vi "Test SimpleDependencyInspector API.vi"() -> ()   [LabVIEW 2019]
doc: "SimpleDependencyInspector API Tester."
uses:
  <vilib>/Utility/error.llb/DialogType.ctl
  arrow color--enum.ctl
  shape--enum.ctl
  SimpleDependencyInspector.lvlib
panel:
  in  "pattern":string[](array[string])=["*.lvlib", "*.lvclass"]
  out "Server Status":bool
  in  "Include vi.lib":bool
  in  "Folder to Inspect":path[](array[path])
  in  "Inspect Project Dependencies":bool
  out "last error":errorcluster
  in  "Show Diagram on Init":bool
  in  "Show Block Diagram":bool
  in  "Stop Module":bool
  in  "Start Module":bool
  in  "Hide Module Panel":bool
  in  "Show Module Panel":bool
  out "Status":string
  out "Module Running?":bool
  # "This VI tests the API for the Module."
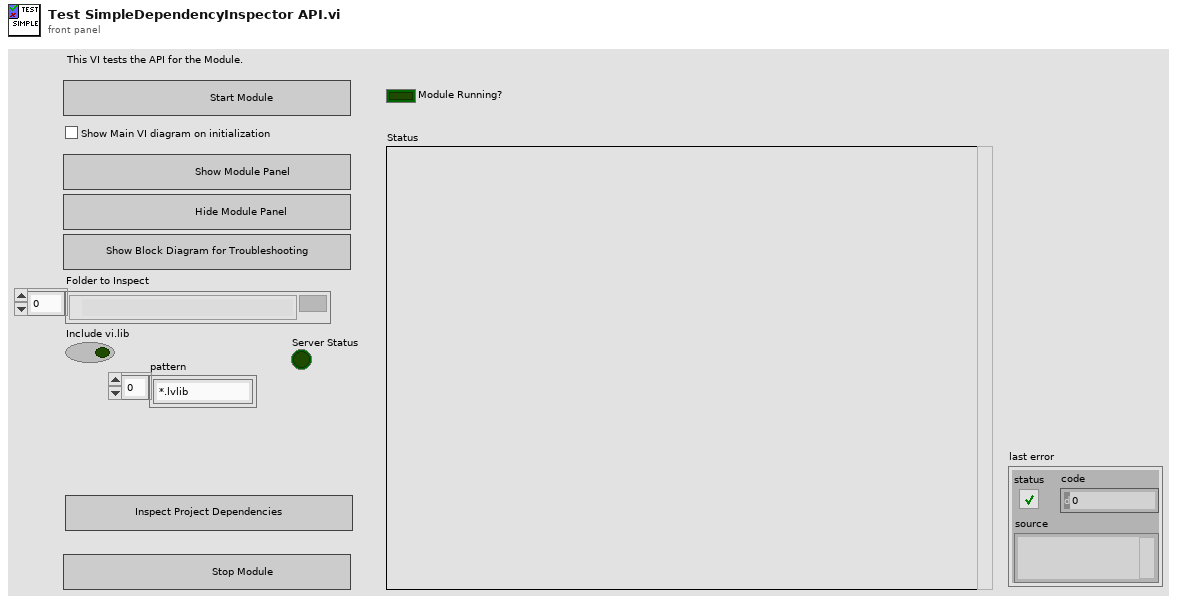
[diagram p1: front panel]
types:
  T1 = typedef "SimpleDependencyInspector.lvlib/Broadcast Events--cluster.ctl" = cluster{"Module Did Init":refnum<user-event>, "Status Updated":refnum<user-event>, "Error Reported":refnum<user-event>, "Module Did Stop":refnum<user-event>, "Update Module Execution Status":refnum<user-event>, "Server Status Updated":refnum<user-event>}
  T2 = typedef "SimpleDependencyInspector.lvlib/shape--enum.ctl" = enum16{"diamond", "triangle", "plaintext", "record", "cylinder", "hexagon", "pentagon", "octagon", "doubleoctagon", "tripleoctagon", "oval", "parallelogram", "point", "egg", "folder", "note", "tab", "terminator", "cds", "trapezium"}
  T3 = typedef "SimpleDependencyInspector.lvlib/arrow color--enum.ctl" = enum16{"random", "green", "red", "yellow", "black", "orange", "blue"}
  T4 = typedef "DialogType.ctl" = u16
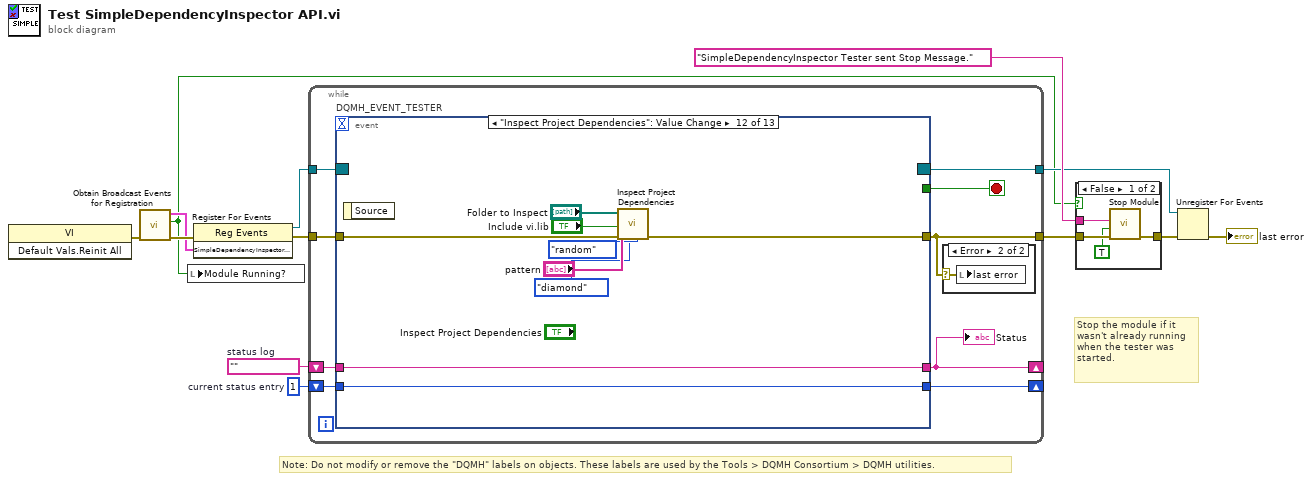
[diagram p0: block diagram]
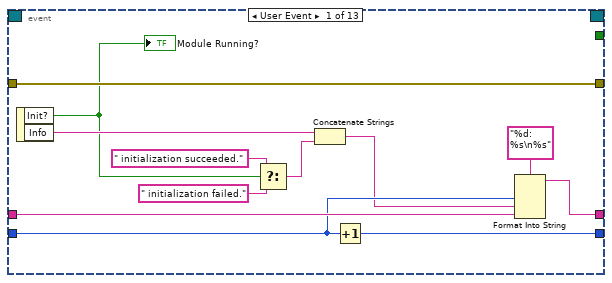
[diagram p4: hidden frame]
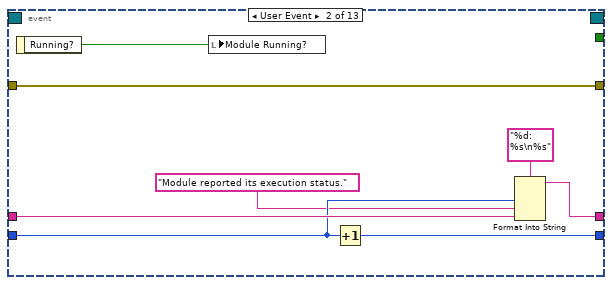
[diagram p5: hidden frame]
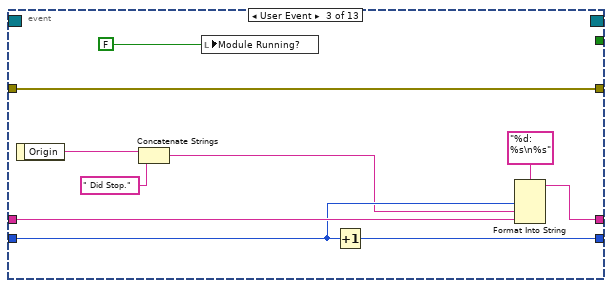
[diagram p6: hidden frame]
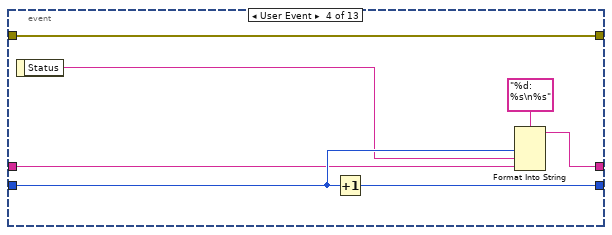
[diagram p7: hidden frame]
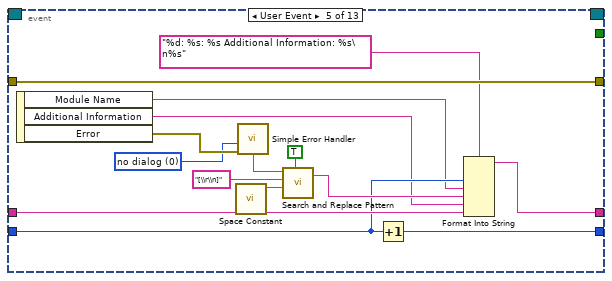
[diagram p8: hidden frame]
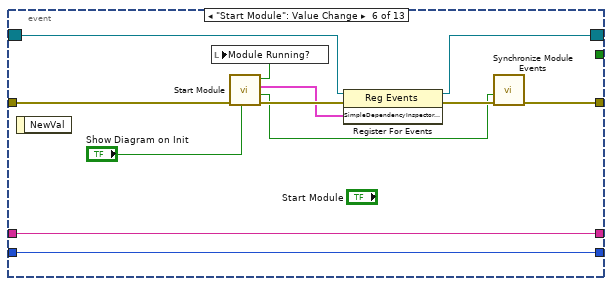
[diagram p9: hidden frame]
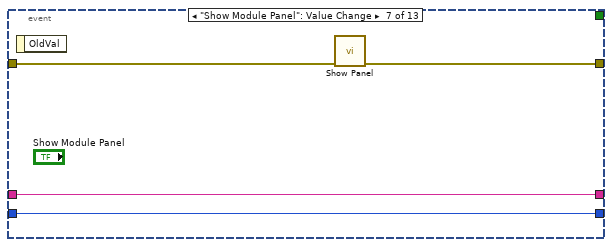
[diagram p10: hidden frame]
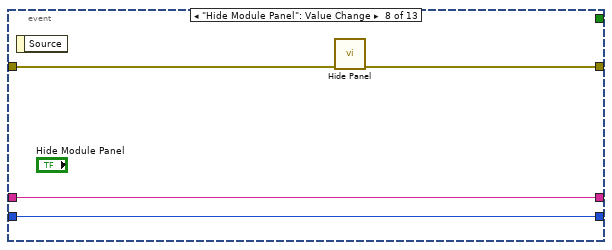
[diagram p11: hidden frame]
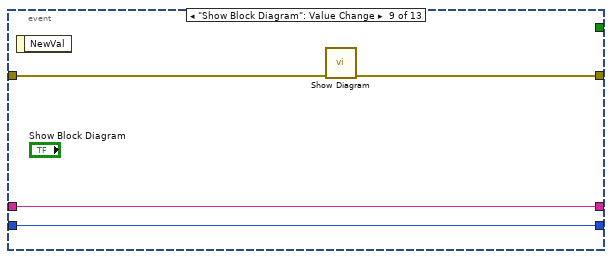
[diagram p12: hidden frame]
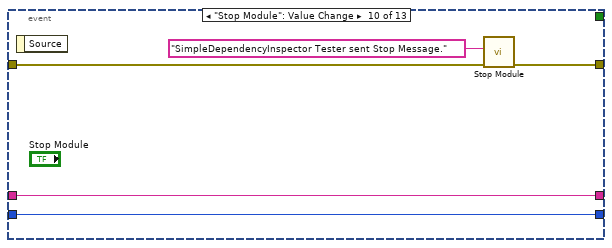
[diagram p13: hidden frame]
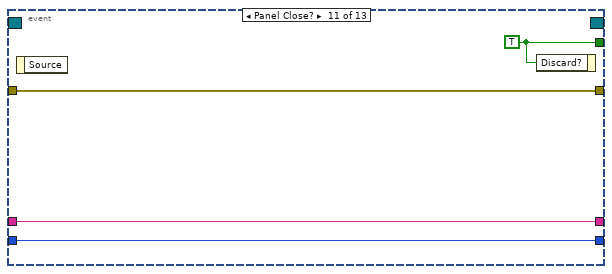
[diagram p14: hidden frame]
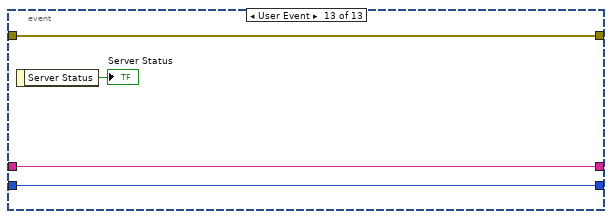
[diagram p15: hidden frame]
diagram:
  w5 = 1  # current status entry
  w6 = ""  # status log
  # "Stop the module if it wasn't already running when the tester was started."
  # "Note: Do not modify or remove the \"DQMH\" labels on objects. These labels are used by the Tools > DQMH Consortium > DQMH utilities."
  n1 = invoke class="VI" method="Default Vals.Reinit All"() -> (error out=w11:errorcluster)  [unwired: 3 in, 2 out]
  n2 = call "Obtain Broadcast Events for Registration.vi"("error in"=w11) -> ("error out"=w10:errorcluster, "Already running?"=w1:bool, "SimpleDependencyInspector Broadcast Events"=w4:T1)  [unwired: 8 in]
  n3 = local write "Module Running?"(w1) -> ()
  n4 = register-events(error in=w10, w4) -> (reference out=w3:refnum<event-registration>, error out=w12:errorcluster)  [unwired: 1 in]
  n5 = while {
    tunnel: w3 -> [w20]
    tunnel: [w21] -> w9
    shift-right: [w16] -> _
    shift-left: w6 -> [w18]
    shift-right: [w17] -> _
    shift-left: w5 -> [w19]
    tunnel: w12 -> [w22]
    tunnel: [w15] -> w2
    stop <- w14 stop-if-true
    n6 = event "DQMH_EVENT_TESTER" shown="[11] \"Inspect Project Dependencies\": Value Change" {
      selector: w20 -> [_ _ _ _ _ w79 _ _ _ _ _ _ _]
      dyn-events: [_ _ _ _ _ w78 _ _ _ _ _ _ _] -> w15
      timeout: _ -> [_ _ _ _ _ _ _ _ _ _ _ _ _]
      tunnel: [_ _ _ _ _ _ _ _ _ _ w107 _ _] -> w14
      tunnel: [w35 w43 w53 w60 w75 w85 w91 w95 w98 w104 w108 w116 w121] -> w21
      tunnel: w19 -> [w32 w40 w50 w56 w65 w82 w88 w92 w96 w101 w105 w114 w119]
      tunnel: w18 -> [w33 w41 w51 w55 w66 w83 w89 w93 w97 w102 w106 w115 w120]
      tunnel: [w30 w38 w48 w57 w64 w83 w89 w93 w97 w102 w106 w115 w120] -> w16
      tunnel: [w31 w39 w49 w59 w63 w82 w88 w92 w96 w101 w105 w114 w119] -> w17
      tunnel: w22 -> [w35 w43 w53 w60 w75 w84 w90 w94 w99 w103 w108 w117 w121]
      event User Event {
        n7 = event-data() -> ("Init?"=w27:bool, "Info"=w29:string)  [unwired: 1 in]
        "Module Running?" <- w27
        n8 = Select(t=" initialization succeeded.", s=w27, f=" initialization failed.") -> (s? t:f=w24:string)
        n9 = Concatenate Strings(w29, w24) -> (w28:string)
        n10 = Increment(x=w32) -> (x+1=w31:i32)
        n11 = Format Into String(format string="%d: %s\n%s", w32, w28, w33) -> (resulting string=w30:string)  [unwired: 2 in, 1 out]
      }
      event User Event {
        n12 = event-data() -> ("Running?"=w36:bool)  [unwired: 1 in]
        n13 = local write "Module Running?"(w36) -> ()
        n14 = Increment(x=w40) -> (x+1=w39:i32)
        n15 = Format Into String(format string="%d: %s\n%s", w40, "Module reported its execution status.", w41) -> (resulting string=w38:string)  [unwired: 2 in, 1 out]
      }
      event User Event {
        n16 = event-data() -> ("Origin"=w47:string)  [unwired: 1 in]
        n17 = Concatenate Strings(w47, " Did Stop.") -> (w46:string)
        n18 = local write "Module Running?"(FALSE ("Module Did Init?")) -> ()
        n19 = Increment(x=w50) -> (x+1=w49:i32)
        n20 = Format Into String(format string="%d: %s\n%s", w50, w46, w51) -> (resulting string=w48:string)  [unwired: 2 in, 1 out]
      }
      event User Event {
        n21 = event-data() -> ("Status"=w54:string)  [unwired: 1 in]
        n22 = Increment(x=w56) -> (x+1=w59:i32)
        n23 = Format Into String(format string="%d: %s\n%s", w56, w54, w55) -> (resulting string=w57:string)  [unwired: 2 in, 1 out]
      }
      event User Event {
        w67 = T4 0 items=["no dialog", "OK message", "continue or stop message", "OK message + warnings", "continue/stop + warnings"] ("type of dialog (OK msg:1)")
        n24 = event-data() -> ("Module Name"=w62:string, "Additional Information"=w61:string, "Error"=w74:errorcluster)  [unwired: 1 in]
        n25 = call <vilib>:"Space Constant.vi"() -> ("String"=w71:string)
        n26 = call <vilib>:"Simple Error Handler.vi"("type of dialog (OK msg:1)"=w67, "error in (no error)"=w74) -> ("message"=w68:string)  [unwired: 3 in, 4 out]
        n27 = call <vilib>:"Search and Replace Pattern.vi"("string"=w68, "regular expression (\"\")"="[\\r\\n]" ("regular expression (\"\")"), "replace string (\"\")"=w71, "replace all? (F)"=TRUE ("replace all CR/LF with spaces")) -> ("result string"=w69:string)  [unwired: 1 in, 1 out]
        n28 = Increment(x=w65) -> (x+1=w63:i32)
        n29 = Format Into String(format string="%d: %s: %s Additional Information: %s\n%s", w65, w62, w69, w61, w66) -> (resulting string=w64:string)  [unwired: 2 in, 1 out]
      }
      event "Start Module": Value Change {
        n30 = event-data() -> ()  [unwired: 1 in, 1 out]
        n31 = call "Start Module.vi"("Show Main VI Diagram on Init (F)"="Show Diagram on Init", "error in"=w84) -> ("error out"=w86:errorcluster, "Wait for Event Sync?"=w81:bool, "SimpleDependencyInspector Broadcast Events"=w80:T1, "Module Was Already Running?"=w77:bool)  [unwired: 6 in]
        n32 = local write "Module Running?"(w77) -> ()
        n33 = register-events(reference=w79, error in=w86, w80) -> (reference out=w78:refnum<event-registration>, error out=w87:errorcluster)
        n34 = call "Synchronize Module Events.vi"("error in"=w87, "Wait for Event Sync?"=w81) -> ("error out"=w85:errorcluster)  [unwired: 9 in]
      }
      event "Show Module Panel": Value Change {
        n35 = event-data() -> ()  [unwired: 1 in, 1 out]
        n36 = call "Show Panel.vi"("error in"=w90) -> ("error out"=w91:errorcluster)  [unwired: 10 in]
      }
      event "Hide Module Panel": Value Change {
        n37 = event-data() -> ()  [unwired: 1 in, 1 out]
        n38 = call "Hide Panel.vi"("error in"=w94) -> ("error out"=w95:errorcluster)  [unwired: 10 in]
      }
      event "Show Block Diagram": Value Change {
        n39 = event-data() -> ()  [unwired: 1 in, 1 out]
        n40 = call "Show Diagram.vi"("error in"=w99) -> ("error out"=w98:errorcluster)  [unwired: 10 in]
      }
      event "Stop Module": Value Change {
        n41 = event-data() -> ()  [unwired: 1 in, 1 out]
        n42 = call "Stop Module.vi"("error in"=w103, "Origin"="SimpleDependencyInspector Tester sent Stop Message.") -> ("error out"=w104:errorcluster)  [unwired: 9 in]
      }
      event Panel Close? {
        w107 = TRUE ("Discard?")
        n43 = event-data() -> ()  [unwired: 1 in, 1 out]
        n44 = event-data("Discard?"=w107) -> ()  [unwired: 1 in, 1 out]
      }
      event "Inspect Project Dependencies": Value Change {
        n45 = event-data() -> ()  [unwired: 1 in, 1 out]
        n46 = call "Inspect Project Dependencies.vi"("Arrow Color"=arrow_color--enum."random", "shape"=shape--enum."diamond", "error in"=w117, "pattern"="pattern", "Include vi.lib"="Include vi.lib", "Path(s) Selection"="Folder to Inspect") -> ("error out"=w116:errorcluster)  [unwired: 5 in]
      }
      event User Event {
        n47 = event-data() -> ("Server Status"=→"Server Status":bool)  [unwired: 1 in]
      }
    }
    "Status" <- w16
    n48 = case shown="Error" w21 {
      selector: w21 -> [_ w23]
      frame No Error {
      }
      frame Error {
        n49 = local write "last error"(w23) -> ()
      }
    }
  }
  n50 = case shown="False" w1 {
    tunnel: [w125 w126] -> w13
    tunnel: "SimpleDependencyInspector Tester sent Stop Message." ("Origin") -> [w123 _]
    tunnel: w9 -> [w124 w126]
    frame False {
      n51 = call "Stop Module.vi"("error in"=w124, "Wait for Module to Stop? (F)"=TRUE ("Wait for Module to stop?"), "Origin"=w123) -> ("error out"=w125:errorcluster)  [unwired: 8 in]
    }
    frame True {
    }
  }
  n52 = Unregister For Events(event registration refnum=w2, error in=w13) -> (error out=→"last error":errorcluster)
